vi "PH_PLH-AccessInformation.panel.vi"(0 "object ref":refnum<vi>, 5 "error in (no error)":errorcluster) -> (19 "error out":errorcluster)   [LabVIEW 2014, in "PH_PLH-AccessInformation.lvlib"]
doc: "By this VI a hardware switch can be monitored and switched. \n\nThe indicators \"FALSE\", \"TRUE\" and \"SWITCH STATE\" show the value of the Beckhoff-Tag: blue indicates bad tag status reference problems, darkgreen false and lightgreen true. If everything is working fine, \"FALSE\" and \"SWITCH STATE\" should show the same value, while \"TRUE\" has the opposite value. The caption of the sensors for \"FALSE\" and \"TRUE\" are taken out of the database. In case of only one or no sensor these GUI elements are not shown at all.\n\nThe oval button switches. It should be in the same state as the \"SWITCH STATE\" indicator. \n\n\"Delete Instance\" disconnects and removes the instance from the PCS.\n\n\nLicense Agreement for this software:\n\nCopyright (C)\nGesellschaft für Schwerionenforschung, GSI\nPlanckstr. 1\n64291 Darmstadt\nGermany\n\nContact: D.Beck@gsi.de \n\nThis program is free software; you can redistribute it and/or modify it under the terms of the GNU General Public License as published by the Free Software Foundation; either version 2 of the license, or (at your option) any later version.\n\nThis program is distributed in the hope that it will be useful, but WITHOUT ANYW ARRANTY; without even the implied warranty of MERCHANTABILITY or FITNESS FOR A PARTICULAR PURPOSE. See the GNU General License for more details (http://www.gnu.org).\n\nGesellschaft für Schwerionenforschung, GSI\nPlanckstr. 1, 64291 Darmstadt, Germany\nFor all questions and ideas contact: M.Richter@gsi.de, H.Brand@gsi.de or D.Beck@gsi.de.\nLast update: 18-DEC-2002"
uses:
  PH_PLH-AccessInformation.lvlib
  CS_Core/CSObj/CSObj.lvlib
  PH_Basics/PH_Common/PH_Common.lvlib
  PH_Basics/PH_Class/PH_Class.lvlib
panel:
  in  "Searchmode":i32(ring) caption="Enabling State" items=["Searchmode: no info", "no Searchmode", "Searchmode"]
  in  "Shotmode":i32(ring) caption="Enabling State" items=["Shotmode: no info", "no Shotmode", "Shotmode"]
  in  "Exit":bool
  in  "Delete":bool
  # "PCS"
  # "3.40"
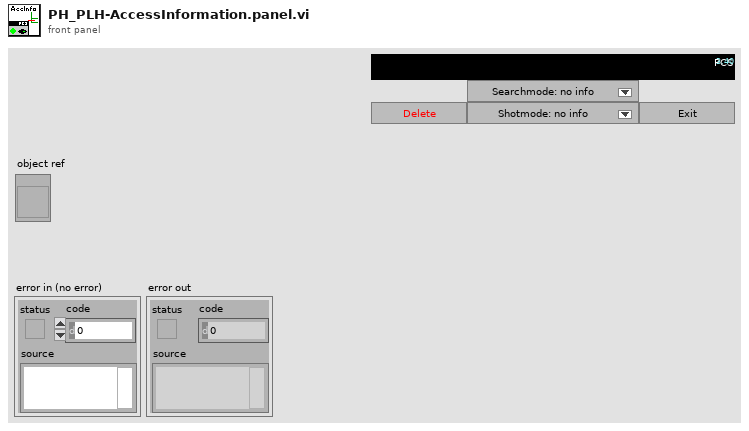
[diagram p1: front panel]
types:
  T1 = typedef "PH_PLH-AccessInformation.lvlib/PH_PLH-AccessInformation.i attribute.ctl" = cluster{"GUI Refs":cluster{"Ref Shotmode":refnum<vi>, "Ref Searchmode":refnum<vi>}, "Shotmode":i32, "Searchmode":i32}
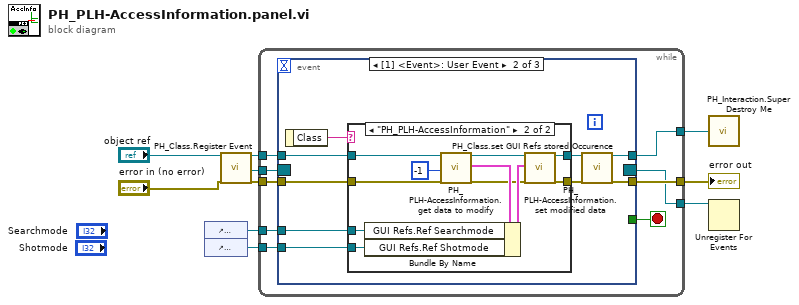
[diagram p0: block diagram]
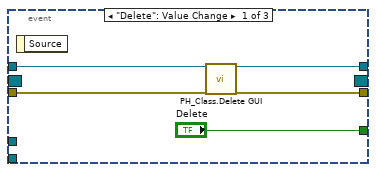
[diagram p2: hidden frame]
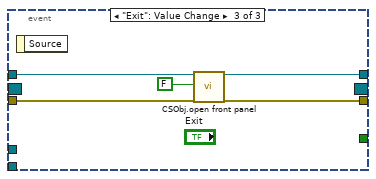
[diagram p4: hidden frame]
diagram:
  n1 = control-ref of="Searchmode"() -> (w4:refnum<vi>)
  n2 = control-ref of="Shotmode"() -> (w3:refnum<vi>)
  n3 = call "PH_Class.Register Event.vi"("i ref in"="object ref", "error in (no error)"="error in (no error)") -> ("i ref out"=w8:refnum<vi>, "Event Registration Refnum"=w6:refnum<event-registration>, "error out"=w7:errorcluster)  [unwired: 15 in]
  n4 = while {
    tunnel: w8 -> [w17]
    tunnel: [w16] -> w10
    tunnel: w7 -> [w19]
    tunnel: [w18] -> w9
    tunnel: w6 -> [w14]
    tunnel: [w13] -> w5
    tunnel: w4 -> [w12]
    tunnel: w3 -> [w11]
    stop <- w15 stop-if-true
    n5 = event shown="[1] <Event>: User Event" {
      selector: w14 -> [_ _ _]
      dyn-events: [_ _ _] -> w13
      timeout: _ -> [_ _ _]
      tunnel: w17 -> [w24 w33 w50]
      tunnel: w19 -> [w23 w31 w49]
      tunnel: [w22 w29 w48] -> w18
      tunnel: [w21 w28 w47] -> w16
      tunnel: ["Delete" _ _] -> w15
      tunnel: w12 -> [_ w27 _]
      tunnel: w11 -> [_ w26 _]
      event "Delete": Value Change {
        n6 = event-data() -> ()  [unwired: 1 in, 1 out]
        n7 = call "PH_Class.Delete GUI.vi"("VI in"=w24, "error in (no error)"=w23) -> ("VI out"=w21:refnum<vi>, "error out"=w22:errorcluster)  [unwired: 16 in]
      }
      event User Event {
        n8 = event-data() -> ("Class"=w25:string)  [unwired: 1 in]
        n9 = case shown="\"PH_PLH-AccessInformation\"" w25 {
          tunnel: w33 -> [w35 w41]
          tunnel: [w35 w40] -> w32
          tunnel: w31 -> [w34 w39]
          tunnel: [w34 w38] -> w30
          tunnel: w27 -> [_ w37]
          tunnel: w26 -> [_ w36]
          frame Default {
          }
          frame "PH_PLH-AccessInformation" {
            n10 = call "PH_PLH-AccessInformation.get data to modify.vi"("i ref in"=w41, "ms timeout (10000)"=-1, "error in (no error)"=w39) -> ("i ref out"=w42:refnum<vi>, "i attribute"=w45:T1, "error out"=w43:errorcluster)  [unwired: 13 in, 1 out]
            n11 = Bundle By Name(cluster=w45, "GUI Refs.Ref Searchmode"=w37, "GUI Refs.Ref Shotmode"=w36) -> (w46:T1)
            n12 = call "PH_PLH-AccessInformation.set modified data.vi"("i ref in"=w42, "i attribute"=w46, "error in (no error)"=w43) -> ("i ref out"=w40:refnum<vi>, "error out"=w38:errorcluster)  [unwired: 15 in]
          }
        }
        n13 = call "PH_Class.set GUI Refs stored Occurence.vi"("i ref in"=w32, "error in (no error)"=w30) -> ("i ref out"=w28:refnum<vi>, "error out"=w29:errorcluster)  [unwired: 16 in]
      }
      event "Exit": Value Change {
        n14 = event-data() -> ()  [unwired: 1 in, 1 out]
        n15 = call "CSObj.open front panel.vi"("i ref in"=w50, "frontPanelOpen"=FALSE ("front panel open"), "error in (no error)"=w49) -> ("i ref out"=w47:refnum<vi>, "error out"=w48:errorcluster)  [unwired: 15 in]
      }
    }
  }
  "error out" <- w9
  n16 = call "PH_Interaction.Super Destroy Me.vi"("i ref out"=w10) -> ()
  n17 = Unregister For Events(event registration refnum=w5) -> ()  [unwired: 1 in, 1 out]
